vi "PicoLog_2.vi"() -> ()   [LabVIEW 2014]
uses:
  picohrdl.dll
panel:
  out "Pico3":dbl(graph)
  out "Over Voltage 3":i16
  in  "Single Ended 3":i16=1 min=0 max=1 step=1
  in  "Conversion 3":i16=3 min=0 max=5 step=1
  in  "Voltage Range 3":i16 min=0 max=6 step=1
  in  "Channel 3":i16=7 min=1 max=16 step=1
  out "Pico2":dbl(graph)
  out "Over Voltage 2":i16
  in  "Single Ended 2":i16=1 min=0 max=1 step=1
  in  "Conversion 2":i16=3 min=0 max=5 step=1
  in  "Voltage Range 2":i16 min=0 max=6 step=1
  in  "Channel 2":i16=9 min=1 max=16 step=1
  out "Pico1":dbl(graph)
  in  "milliseconds to wait":u32=1000
  in  "stop":bool
  out "Over Voltage":i16
  out "Handle":i16
  in  "Single Ended":i16=1 min=0 max=1 step=1
  in  "Conversion":i16=3 min=0 max=5 step=1
  in  "Voltage Range":i16 min=0 max=6 step=1
  in  "Channel":i16=10 min=1 max=16 step=1
  # "-1        if the unit fails to open\n0         if no unit is found\n>= 1   handle to the device opened"
  # "The channel that will be enabled or disabled.\nADC-20: 1 to 8\nADC-24: 1 to 16"
  # "Non-zero to measure a single-ended voltage.\nZero for a differential voltage."
  # "range Voltage range Availability\n (0)    ±2500 mV        ADC-20 and ADC-24\n (1)    ±1250 mV        ADC-20 and ADC-24\n (2)    ±625 mV          ADC-24 only\n (3)    ±312.5 mV       ADC-24 only\n (4)    ±156.25 mV     ADC-24 only\n (5)    ±78.125 mV     ADC-24 only\n (6)    ±39.0625 mV   ADC-24 only"
  # "conversion Conversion time\n(0)               60 ms\n(1)               100 ms\n(2)               180 ms\n(3)               340 ms\n(4)               660 ms"
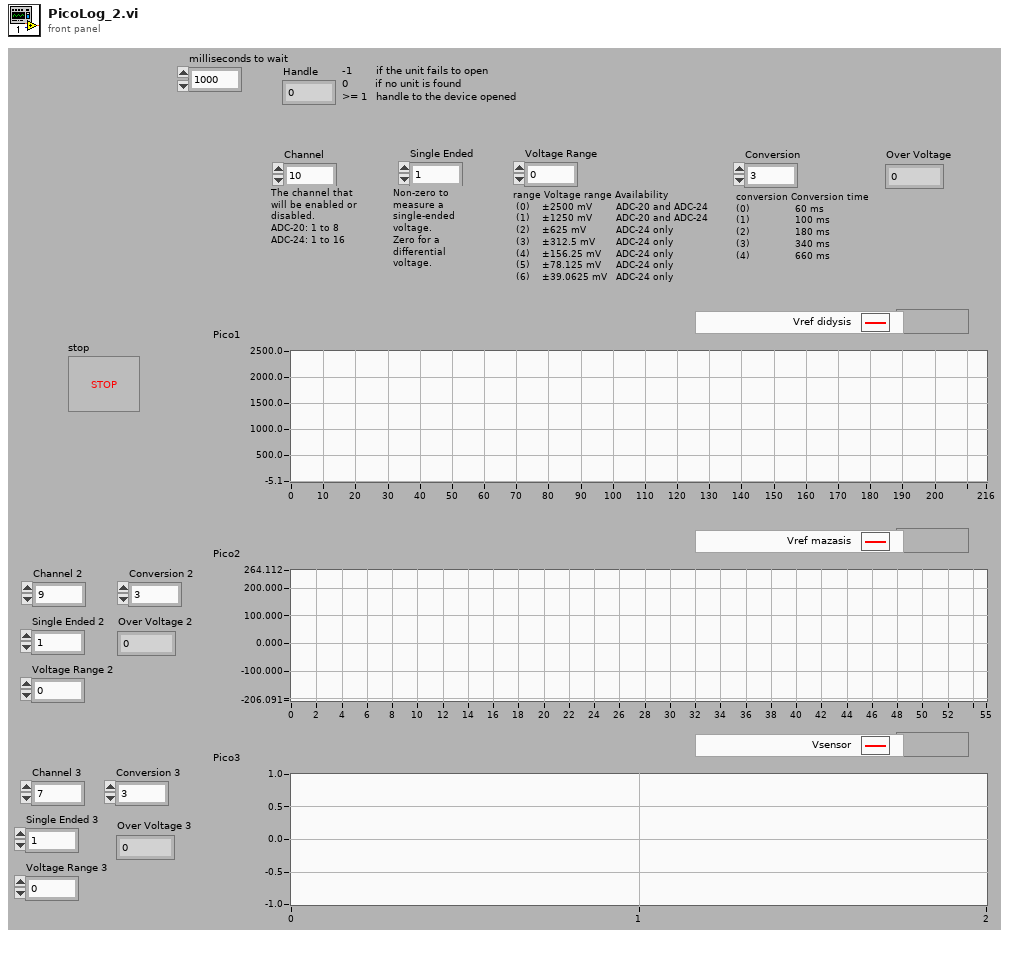
[diagram p1: front panel]
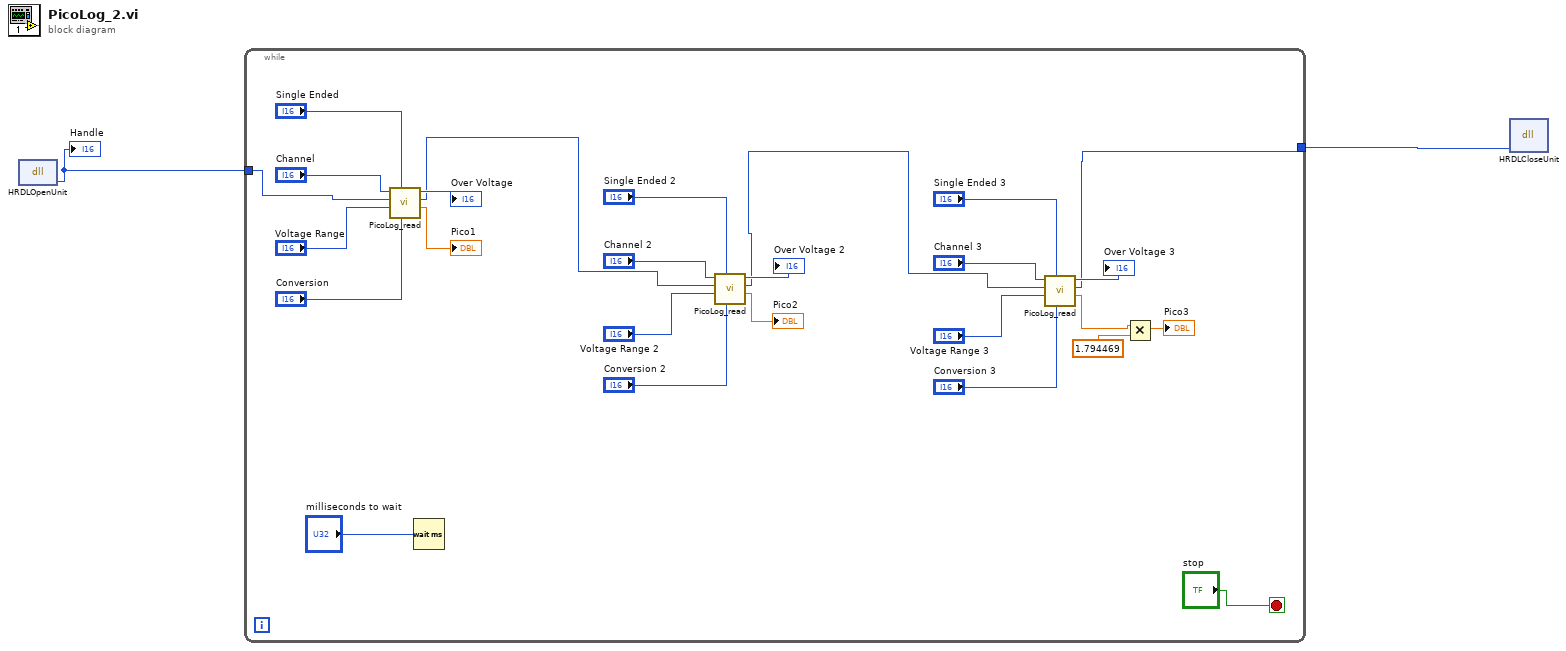
[diagram p0: block diagram]
diagram:
  n1 = dll-call lib="PicoHRDL.dll" fn="HRDLOpenUnit"() -> ("return type"=w2:i16)  [unwired: 3 in, 2 out]
  "Handle" <- w2
  n2 = while {
    tunnel: w2 -> [w26]
    tunnel: [w6] -> w1
    stop <- "stop" stop-if-true
    n3 = call "PicoLog_read.vi"("Conversion"="Conversion", "Single Ended"="Single Ended", "Voltage Range"="Voltage Range", "return type"=w26, "Channel"="Channel") -> ("Numeric"=→"Pico1":dbl, "handle"=w13:i16, "Over Voltage"=→"Over Voltage":i16)  [unwired: 4 in]
    n4 = Wait (ms)(milliseconds to wait="milliseconds to wait") -> ()  [unwired: 1 out]
    n5 = call "PicoLog_read.vi"("Conversion"="Conversion 2", "Single Ended"="Single Ended 2", "Voltage Range"="Voltage Range 2", "return type"=w13, "Channel"="Channel 2") -> ("Numeric"=→"Pico2":dbl, "handle"=w7:i16, "Over Voltage"=→"Over Voltage 2":i16)  [unwired: 4 in]
    n6 = call "PicoLog_read.vi"("Conversion"="Conversion 3", "Single Ended"="Single Ended 3", "Voltage Range"="Voltage Range 3", "return type"=w7, "Channel"="Channel 3") -> ("Numeric"=w5:dbl, "handle"=w6:i16, "Over Voltage"=→"Over Voltage 3":i16)  [unwired: 4 in]
    n7 = Multiply(x=w5, y=1.794469) -> (x*y=→"Pico3":dbl)
  }
  n8 = dll-call lib="PicoHRDL.dll" fn="HRDLCloseUnit"("handle"=w1) -> ()  [unwired: 5 in, 2 out]
